vi "Debug Exercise (Main).vi"() -> ()   [LabVIEW 2025]
doc: "This exercise is used to demonstrate the use of different debugging tools."
panel:
  out "Final Result":dbl format="%.2f"
  out "Random Number":dbl format="%.2f"
  out "Multiply Result":dbl format="%.2f"
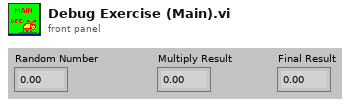
[diagram p1: front panel]
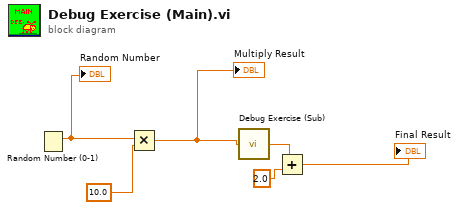
[diagram p0: block diagram]
diagram:
  n1 = Random Number (0-1)() -> (number: 0 to 1=w6:dbl)
  "Random Number" <- w6
  n2 = Multiply(x=w6, y=10.0) -> (x*y=w1:dbl)
  "Multiply Result" <- w1
  n3 = call "Debug Exercise (Sub).vi"("Number"=w1) -> ("Final Result"=w4:dbl)
  n4 = Add(x=w4, y=2.0) -> (x+y=→"Final Result":dbl)
